vi "Get Bitfile Path.vi"(8 "error in (no error)":errorcluster, 10 "SI Count":i32, 11 "Module Name":string) -> (0 "error out":errorcluster, 3 "Bitfile Path":path)   [LabVIEW 2025]
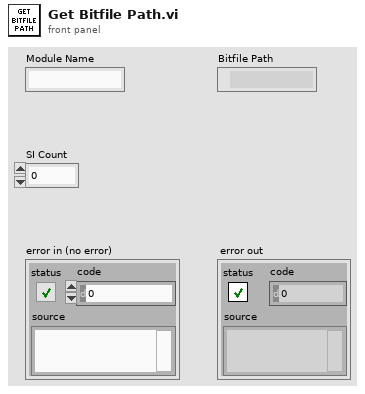
[diagram p1: front panel]
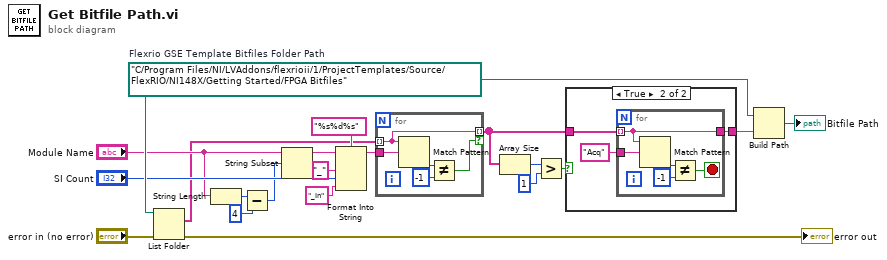
[diagram p0: block diagram]
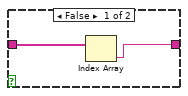
[diagram p2: hidden frame]
diagram:
  w16 = path "C:/Program Files/NI/LVAddons/flexrioii/1/ProjectTemplates/Source/FlexRIO/NI148X/Getting Started/FPGA Bitfiles"  # Flexrio GSE Template Bitfiles Folder Path
  n1 = List Folder(path=w16, error in="error in (no error)") -> (filenames=w1:string[], error out=→"error out":errorcluster)  [unwired: 2 in, 2 out]
  n2 = String Length(string="Module Name") -> (length=w3:i32)
  n3 = Subtract(x=w3, y=4) -> (x-y=w4:i32)
  n4 = String Subset(string="Module Name", offset (0)=w4) -> (substring=w7:string)  [unwired: 1 in]
  n5 = Format Into String(format string="%s%d%s", initial string=w7, "_" ("substring"), "SI Count", "_In" ("substring")) -> (resulting string=w8:string)  [unwired: 1 in, 1 out]
  n6 = for {
    tunnel: w1 -> [w22] mode=indexing
    tunnel: w8 -> [w25]
    tunnel: [w22] -> w15 mode=indexing if=w21
    n7 = Match Pattern(string=w22, regular expression=w25) -> (offset past match=w23:i32)  [unwired: 1 in, 3 out]
    n8 = Not Equal?(x=w23, y=-1) -> (x != y?=w21:bool)
  }
  n9 = Array Size(array=w15) -> (size(s)=w12:i32)
  n10 = Greater?(x=w12, y=1) -> (0:w14:bool)
  n11 = case shown="True" w14 {
    tunnel: w15 -> [w27 w30]
    tunnel: [w26 w28] -> w17
    frame False {
      n12 = Index Array(array=w27) -> (element=w26:string)  [unwired: 1 in]
    }
    frame True {
      n13 = for {
        tunnel: w30 -> [w32] mode=indexing
        tunnel: "Acq" -> [w35]
        tunnel: [w32] -> w28
        stop <- w31 stop-if-true
        n14 = Match Pattern(string=w32, regular expression=w35) -> (offset past match=w33:i32)  [unwired: 1 in, 3 out]
        n15 = Not Equal?(x=w33, y=-1) -> (x != y?=w31:bool)
      }
    }
  }
  n16 = Build Path(base path=w16, name or relative path=w17) -> (appended path=→"Bitfile Path":path)
